vi "pharosReadClose.vi"   [LabVIEW 2017]
uses:
  globalDevices.vi
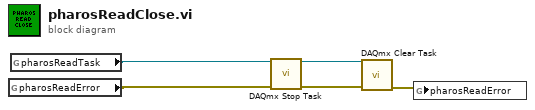
[diagram p0: block diagram]
diagram:
  n1 = global read "globalDevices.vi" "pharosReadError"() -> (w2:errorcluster)
  n2 = global read "globalDevices.vi" "pharosReadTask"() -> (w3:refnum<k21>)
  n3 = call <vilib>:"DAQmx Stop Task.vi"("task/channels in"=w3, "error in"=w2) -> ("task out"=w5:refnum<k21>, "error out"=w4:errorcluster)  [unwired: 12 in]
  n4 = call <vilib>:"DAQmx Clear Task.vi"("task in"=w5, "error in"=w4) -> ("error out"=w1:errorcluster)  [unwired: 13 in]
  n5 = global write "globalDevices.vi" "pharosReadError"(w1) -> ()
